vi "Update I2C Messages Table.vi"(8 "error in (no error)":errorcluster, 10 "I2C Messages in":string[][](array[string]), 11 "Table in":refnum<vi>) -> (0 "error out":errorcluster)   [LabVIEW 2025]
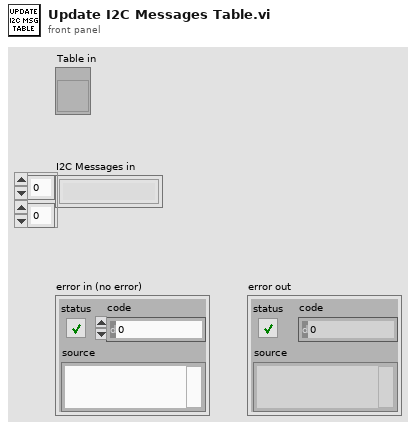
[diagram p1: front panel]
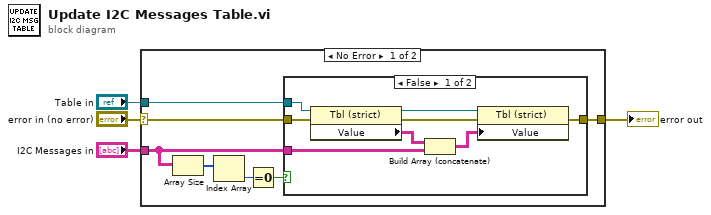
[diagram p0: block diagram]
diagram:
  n1 = case shown="No Error" "error in (no error)" {
    selector: "error in (no error)" -> [w6 w21]
    tunnel: "Table in" -> [w11 _]
    tunnel: "I2C Messages in" -> [w8 _]
    tunnel: [w5 w21] -> w1
    frame No Error {
      n2 = Array Size(array=w8) -> (size(s)=w7:i32[])
      n3 = Index Array(array=w7) -> (element=w9:i32)  [unwired: 1 in]
      n4 = Equal To 0?(x=w9) -> (x = 0?=w10:bool)
      n5 = case shown="False" w10 {
        tunnel: w8 -> [w19 _]
        tunnel: w11 -> [w17 _]
        tunnel: w6 -> [w14 w20]
        tunnel: [w13 w20] -> w5
        frame False {
          n6 = property on="Property Node" class="Tbl (strict)"(reference=w17, error in=w14) -> (reference out=w15:refnum<vi>, error out=w12:errorcluster, "Value"=w16:string[][])
          n7 = Build Array (concatenate)(w16, w19) -> (w18:string[][])
          n8 = property on="Property Node" class="Tbl (strict)"(reference=w15, error in=w12, "Value"=w18) -> (error out=w13:errorcluster)  [unwired: 1 out]
        }
        frame True {
        }
      }
    }
    frame Error {
    }
  }
  "error out" <- w1
